vi "CSV Parsing.vi"() -> (2 "Files in Directory":path[](array[path]), 3 "CSV Data":string[][][](array[string]))   [LabVIEW 2015]
uses:
  <vilib>/Utility/sysdir.llb/System Directory Type.ctl
  <vilib>/Utility/file.llb/Read Delimited Spreadsheet (string).vi
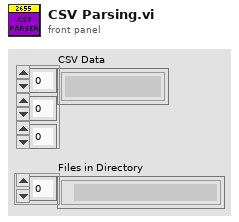
[diagram p1: front panel]
types:
  T1 = typedef "System Directory Type.ctl" = i32
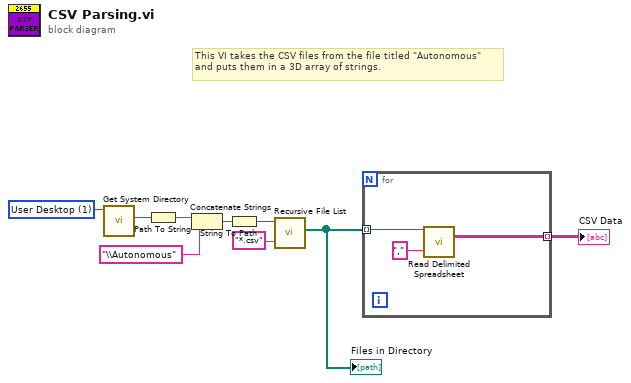
[diagram p0: block diagram]
diagram:
  w6 = T1 1 items=["User Home"=0, "User Desktop"=1, "User Documents"=2, "User Application Data"=3, "User Preferences"=4, "User Temporary"=5, "Public Documents"=6, "Public Application Data"=7, "Public Preferences"=8, "Public Cache"=13, "System Core Libraries"=9, "System Installed Libraries"=10, "Application Files"=11, "Boot Volume Root"=12] ("system directory type")
  # "This VI takes the CSV files from the file titled \"Autonomous\" and puts them in a 3D array of strings."
  n1 = call <vilib>:"Get System Directory.vi"("system directory type"=w6) -> ("system directory"=w5:path)  [unwired: 10 in]
  n2 = Path To String(path=w5) -> (string=w4:string)
  n3 = Concatenate Strings(w4, "\\Autonomous" ("string")) -> (w2:string)
  n4 = String To Path(string=w2) -> (path=w3:path)
  n5 = call <vilib>:"Recursive File List.vi"("pattern"="*.csv", "Folder Path"=w3) -> ("All Files in Dir"=w7:path[])  [unwired: 5 in, 4 out]
  "Files in Directory" <- w7
  n6 = for {
    tunnel: [w11] -> w8 mode=indexing
    tunnel: w7 -> [w10] mode=indexing
    n7 = call-poly <vilib>:"Read Delimited Spreadsheet.vi"("file path (dialog if empty)"=w10, "delimiter (\\t)"="," ("delimiter (\\t)")) -> ("all rows"=w11:string[][])  [unwired: 8 in, 5 out]
  }
  "CSV Data" <- w8
